vi "ADCP_Verify_Checksum_Processed_Packet.vi"(8 "error in (no error)":errorcluster, 10 "Processed Packet":u8[](array[numeric]), 11 "ADCP in":refnum<class "ADCP.lvclass">) -> (0 "error out":errorcluster, 2 "Checksum Valid ?":bool, 3 "ADCP out":refnum<class "ADCP.lvclass">)   [LabVIEW 2017, in "ADCP.lvclass"]
uses:
  ADCP.lvclass
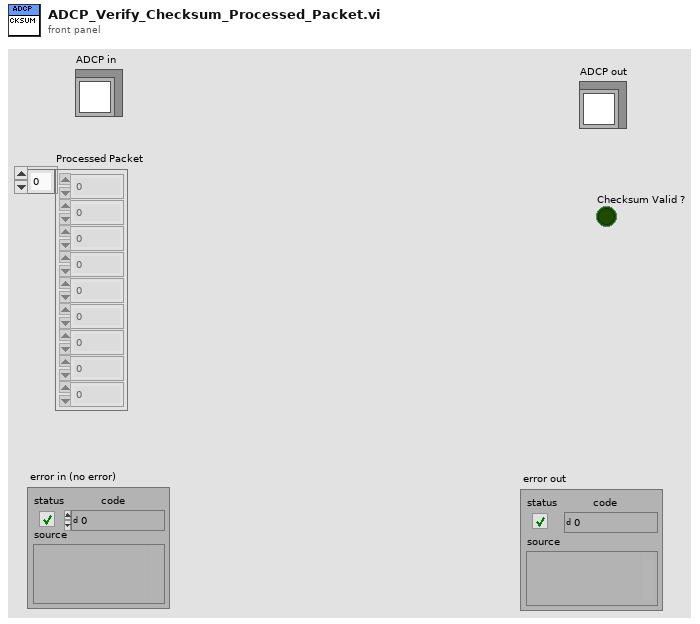
[diagram p1: front panel]
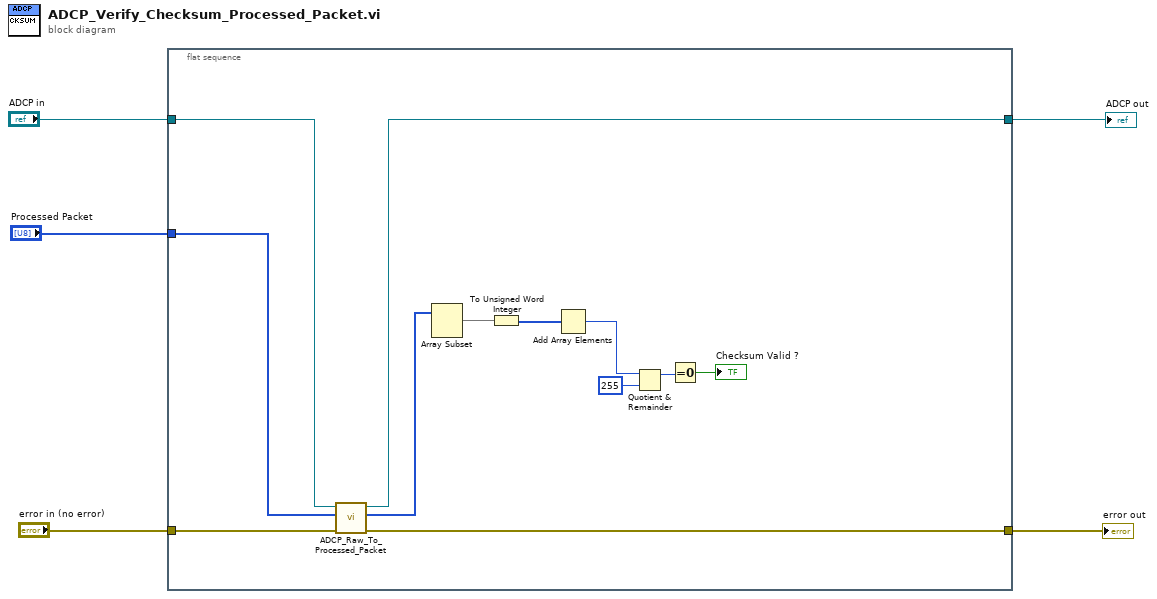
[diagram p0: block diagram]
diagram:
  n1 = flat-sequence {
    tunnel: "ADCP in" -> [w9]
    tunnel: "Processed Packet" -> [w7]
    tunnel: "error in (no error)" -> [w11]
    tunnel: [w8] -> w2
    tunnel: [w10] -> w1
    frame #0 {
      n2 = call "ADCP_Raw_To_Processed_Packet.vi"("error in (no error)"=w11, "Raw Packet"=w7, "ADCP in"=w9) -> ("error out"=w10:errorcluster, "Processed Packet"=w6:u8[], "ADCP out"=w8:refnum<class "ADCP.lvclass">)  [unwired: 6 in]
      n3 = Array Subset(array=w6) -> (w17:u8[])  [unwired: 2 in]
      n4 = To Unsigned Word Integer(number=w17) -> (unsigned 16bit integer=w16:u16[])
      n5 = Add Array Elements(numeric array=w16) -> (sum=w15:u16)
      n6 = Quotient & Remainder(x=w15, y=u16 255) -> (x-y*floor(x/y)=w13:u16)  [unwired: 1 out]
      n7 = Equal To 0?(x=w13) -> (x = 0?=→"Checksum Valid ?":bool)
    }
  }
  "ADCP out" <- w2
  "error out" <- w1
